vi "CreateInputNode.vi"(8 "Error In":errorcluster, 10 "Input":T1, 11 "DOM Document":refnum<k20>) -> (0 "Error Out":errorcluster, 3 "Input Node":refnum<k20>)   [LabVIEW 2012, in "Virtual-PGA.lvlib"]
uses:
  Virtual-PGA.lvlib
  Public/Controls/Input.ctl
  <resource>/objmgr/DOMUserDefRef.rc
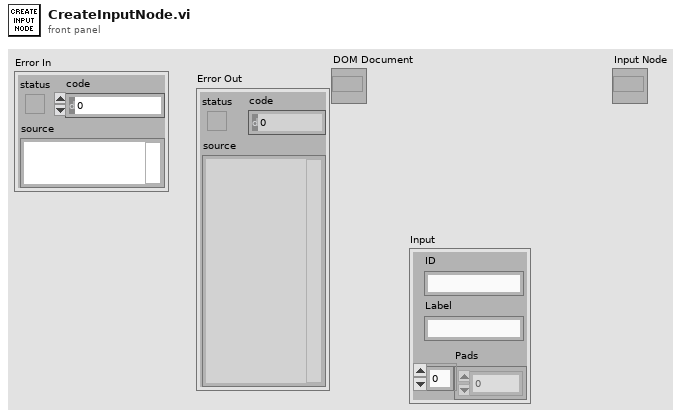
[diagram p1: front panel]
types:
  T1 = typedef "Virtual-PGA.lvlib/Input.ctl" = cluster{"ID":string, "Label":string, "Pads":u32[]}
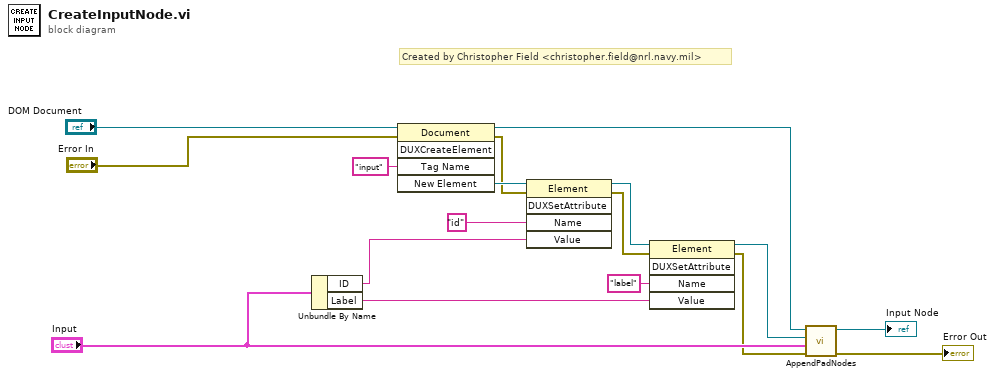
[diagram p0: block diagram]
diagram:
  # "Created by Christopher Field <christopher.field@nrl.navy.mil>"
  n1 = Unbundle By Name("Input") -> ("ID"=w2:string, "Label"=w1:string)
  n2 = invoke class="Document" method="DUXCreateElement"(reference="DOM Document", error in="Error In", "Tag Name"="input") -> (reference out=w5:refnum<k20>, error out=w7:errorcluster, "New Element"=w11:refnum<k20>)  [unwired: 2 in, 2 out]
  n3 = invoke class="Element" method="DUXSetAttribute"(reference=w11, error in=w7, "Name"="id", "Value"=w2) -> (reference out=w9:refnum<k20>, error out=w6:errorcluster)  [unwired: 1 in, 3 out]
  n4 = invoke class="Element" method="DUXSetAttribute"(reference=w9, error in=w6, "Name"="label", "Value"=w1) -> (reference out=w3:refnum<k20>, error out=w4:errorcluster)  [unwired: 1 in, 3 out]
  n5 = call "AppendPadNodes.vi"("Error In"=w4, "Input"="Input", "Input Node In"=w3, "DOM Document"=w5) -> ("Error Out"=→"Error Out":errorcluster, "Input Node Out"=→"Input Node":refnum<k20>)  [unwired: 6 in]
